vi "GetPosSingleAxis.vi"(8 "error in (no error)":errorcluster, 10 "Axis":i32=1 min=1 max=4, 11 "DelayLineSimulation in":refnum<class "DLEmulate.lvclass">) -> (0 "error out":errorcluster, 2 "Pos":dbl, 3 "DelayLineSimulation out":refnum<class "DLEmulate.lvclass">)   [LabVIEW 2019, in "DLEmulate.lvclass"]
uses:
  DLEmulate.lvclass
  DLEmulate.lvclass/DLEmulate.ctl
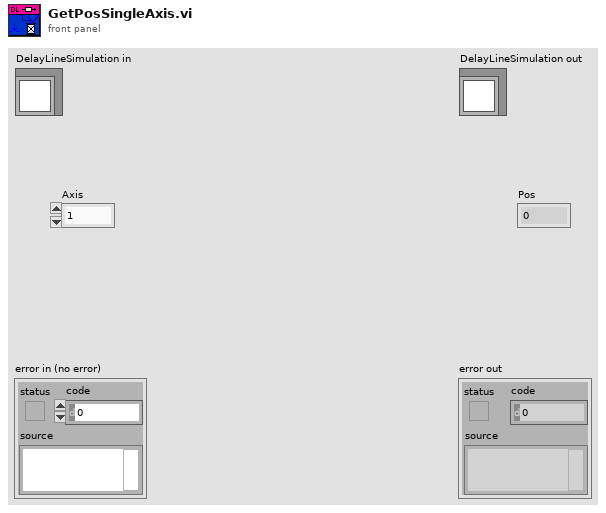
[diagram p1: front panel]
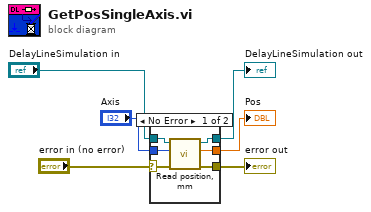
[diagram p0: block diagram]
diagram:
  n1 = case shown="No Error" "error in (no error)" {
    selector: "error in (no error)" -> [w11 w14]
    tunnel: [w8 w14] -> w5
    tunnel: [w9 w13] -> w4
    tunnel: "DelayLineSimulation in" -> [w12 w13]
    tunnel: "Axis" -> [w10 _]
    tunnel: [w7 _] -> w1
    frame No Error {
      n2 = call "Read position, mm.vi"("error in (no error)"=w11, "axis"=w10, "DelayLineSimulation in"=w12) -> ("error out"=w8:errorcluster, "position, mm"=w7:dbl, "DelayLineSimulation out"=w9:refnum<class "DLEmulate.lvclass">)  [unwired: 6 in]
    }
    frame Error {
    }
  }
  "error out" <- w5
  "DelayLineSimulation out" <- w4
  "Pos" <- w1
